vi "Frequency9225-7_FPGA.vi"(1 "dF [Hz]":fxp<+,36,5>=12.20703125, 2 "dBin [-0.5,0.5)":fxp<+/-,36,0>, 3 "iMAX":u16) -> (0 "Frequency [Hz]":fxp<+,36,7>)   [LabVIEW 2021]
uses:
  <vilib>/rvi/FXPMathLib/FxpAdd/XNode/nifxpmath_Add.xnode
  <vilib>/rvi/FXPMathLib/sim/FxpSim.dll
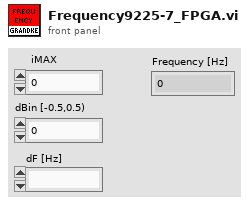
[diagram p1: front panel]
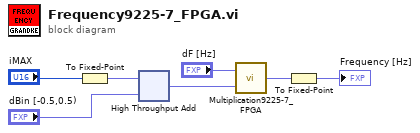
[diagram p0: block diagram]
diagram:
  n1 = To Fixed-Point(number="iMAX") -> (fixed-point=w7:fxp<+,16,16>)  [unwired: 1 in]
  n2 = xnode "High Throughput Add"("x"=w7, "y"="dBin [-0.5,0.5)") -> ("x+y"=w3:fxp<+,36,3>)
  n3 = call "Multiplication9225-7_FPGA.vi"("y <+/-44,8>"=w3, "x <+/-47,6>"="dF [Hz]") -> ("x*y <+/-49,13>"=w5:fxp<+/-,49,13>)
  n4 = To Fixed-Point(number=w5) -> (fixed-point=→"Frequency [Hz]":fxp<+,36,7>)  [unwired: 1 in]
